vi "Set Mode.vi"(6 "Channel":i32=1, 8 "error in (no error)":errorcluster, 10 "Waveform":T1, 11 "336XX in":refnum<class "336XX.lvclass">) -> (0 "error out":errorcluster, 3 "336XX out":refnum<class "336XX.lvclass">)   [LabVIEW 2019, in "336XX.lvlib" / "336XX.lvclass"]
uses:
  Library/336XX.lvclass
  builds/Instruments/FunctionGenerator.lvlibp/Custom Controls/WaveformMode.ctl
  builds/Instruments/FunctionGenerator.lvlibp/Library/FunctionGenerator.lvclass
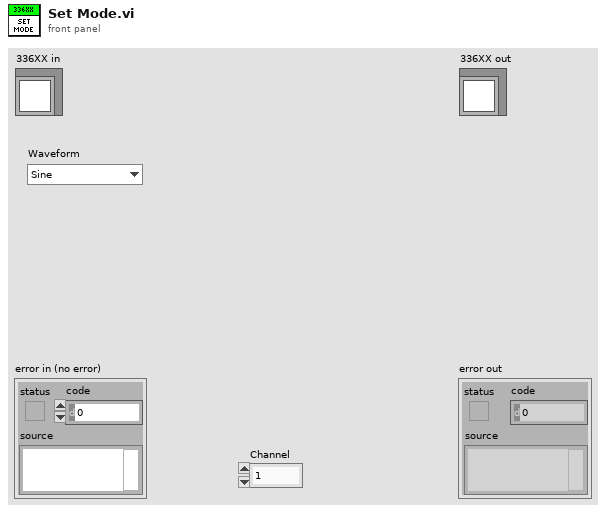
[diagram p1: front panel]
types:
  T1 = typedef "FunctionGenerator.lvlibp/FunctionGenerator.lvclass/WaveformMode.ctl" = enum16{"Sine", "Square", "Ramp", "Pulse", "Arbitrary", "Triangle", "Noise", "DC"}
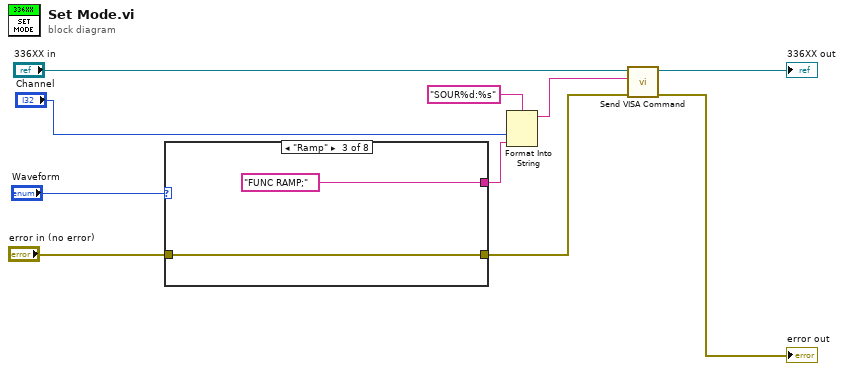
[diagram p0: block diagram]
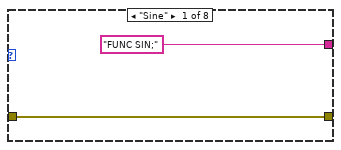
[diagram p2: hidden frame]
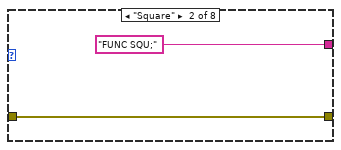
[diagram p3: hidden frame]
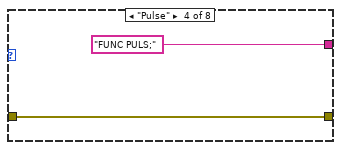
[diagram p4: hidden frame]
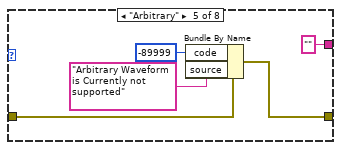
[diagram p5: hidden frame]
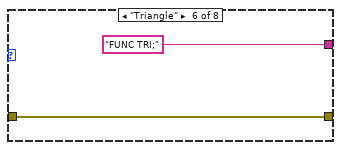
[diagram p6: hidden frame]
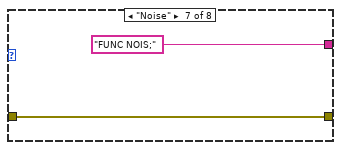
[diagram p7: hidden frame]
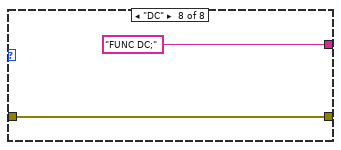
[diagram p8: hidden frame]
diagram:
  n1 = case shown="\"Ramp\"" "Waveform" {
    tunnel: ["FUNC SIN;" ("format string") "FUNC SQU;" ("format string") "FUNC RAMP;" ("format string") "FUNC PULS;" ("format string") "" ("format string") "FUNC TRI;" ("format string") "FUNC NOIS;" ("format string") "FUNC DC;" ("format string")] -> w2
    tunnel: "error in (no error)" -> [w11 w13 w15 w17 w23 w24 w26 w28]
    tunnel: [w11 w13 w15 w17 w21 w24 w26 w28] -> w5
    frame "Sine" {
    }
    frame "Square" {
    }
    frame "Ramp" {
    }
    frame "Pulse" {
    }
    frame "Arbitrary" {
      n2 = Bundle By Name(cluster=w23, "code"=-89999, "source"="Arbitrary Waveform is Currently not supported") -> (w21:errorcluster)
    }
    frame "Triangle" {
    }
    frame "Noise" {
    }
    frame "DC" {
    }
  }
  n3 = Format Into String(format string="SOUR%d:%s", "Channel", w2) -> (resulting string=w1:string)  [unwired: 2 in, 1 out]
  n4 = call "Send VISA Command.vi"("error in (no error)"=w5, "Command"=w1, "336XX in"="336XX in") -> ("error out"=→"error out":errorcluster, "336XX out"=→"336XX out":refnum<class "336XX.lvclass">)  [unwired: 7 in]
